vi "generalParameters_init.vi"() -> (3 "General Parameters":T1)   [LabVIEW 2013]
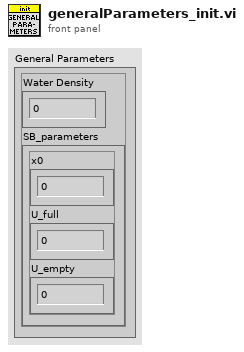
[diagram p1: front panel]
types:
  T1 = cluster{"Water Density":dbl, "SB_parameters":cluster{"x0":dbl, "U_full":dbl, "U_empty":dbl}}
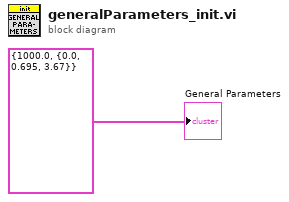
[diagram p0: block diagram]
diagram:
  "General Parameters" <- T1 {"Water Density"=1000.0, "SB_parameters"={"x0"=0.0, "U_full"=0.695, "U_empty"=3.67}}
